vi "Drive.vi"   [LabVIEW 2018]
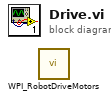
[diagram p0: block diagram]
diagram:
  n1 = call <vilib>:"WPI_RobotDriveMotors.vi"() -> ()  [unwired: 9 in, 3 out]
